vi "Change Function.vi"(8 "error in (no error)":errorcluster, 9 "Measurement Rate (0: Slow)":u16(ring) items=["Slow", "Medium", "Fast"], 10 "Measurement Function (0: DC Volts)":u16(ring) items=["DC Volts", "AC Volts", "DC Current", "AC Current", "2-Wire Resistance", "4-Wire Resistance", "Frequency", "AC and DC rms Current", "AC and DC rms Volts", "Continuity", "Diode"], 11 "Tektronix DMM4020 in":refnum<class "Tektronix DMM4020.lvclass">) -> (0 "error out":errorcluster, 3 "Tektronix DMM4020 out":refnum<class "Tektronix DMM4020.lvclass">)   [LabVIEW 2016, in "Generic Digital Multi Meter.lvlib" / "Tektronix DMM4020.lvlib" / "Tektronix DMM4020.lvclass"]
uses:
  Tektronix DMM4020.lvclass
  <instrlib>/Tektronix DMM4020/Tektronix DMM4020.lvlib
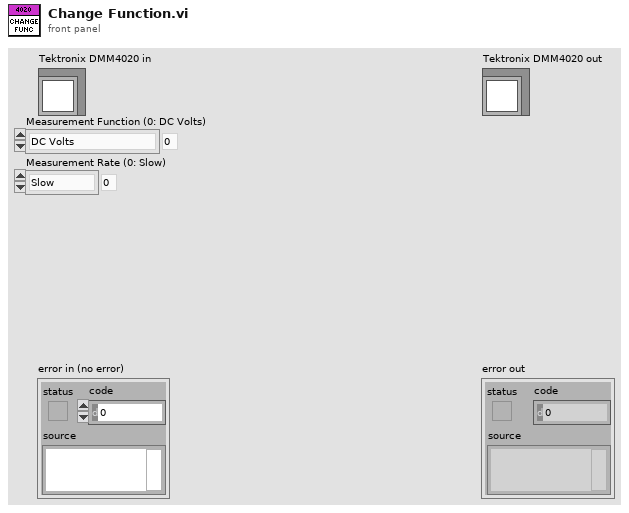
[diagram p1: front panel]
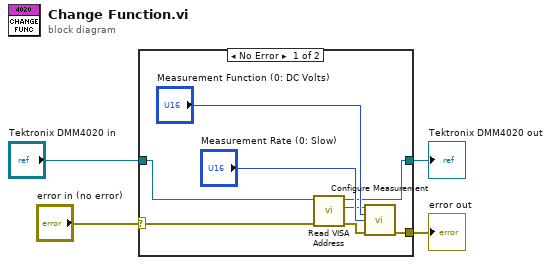
[diagram p0: block diagram]
diagram:
  n1 = case shown="No Error" "error in (no error)" {
    selector: "error in (no error)" -> [w8 w14]
    tunnel: [w12 w14] -> w3
    tunnel: [w6 w13] -> w1
    tunnel: "Tektronix DMM4020 in" -> [w9 w13]
    frame No Error {
      n2 = call-dynamic "Read VISA Address.vi"("error in (no error)"=w8, "Generic Device in"=w9) -> ("error out"=w7:errorcluster, "VISA Address"=w5:refnum<visa-resource-name>, "Generic Device out"=w6:refnum<class "Tektronix DMM4020.lvclass">)  [unwired: 7 in]
      n3 = call <instrlib>:"Configure Measurement.vi"("VISA resource name"=w5, "Measurement Function (0: DC Volts)"="Measurement Function (0: DC Volts)", "Measurement Rate (0: Slow)"="Measurement Rate (0: Slow)", "error in (no error)"=w7) -> ("error out"=w12:errorcluster)  [unwired: 10 in, 1 out]
    }
    frame Error {
    }
  }
  "error out" <- w3
  "Tektronix DMM4020 out" <- w1
